vi "PH_PPPA_PowerUnit.PC_StateIgni.vi"(0 "i ref in":refnum<vi>, 3 "Igni Status":T1 items=["no info", "off/false/out", "on/true/in", "Failure", "Alarm", "Status 1", "Status 2", "Status 3"], 4 "not linked?":bool, 5 "error in (no error)":errorcluster) -> (14 "i ref out":refnum<vi>, 19 "error out":errorcluster)   [LabVIEW 2014, in "PH_PPPA_PowerUnit.lvlib"]
doc: "This VI writes the Ignitron Tag values to own attributes, calculates the state of the device and sets the GUI object."
uses:
  PH_PPPA_PowerUnit.lvlib
  PH_StatusHandler/PH_StatusHandler.Status.ctl
  PH_Common/PH_Common.lvlib
  PH_PowerUnit_BaseClass/PH_PowerUnit_BaseClass.lvlib
  PH_StatusHandler/PH_StatusHandler.lvlib
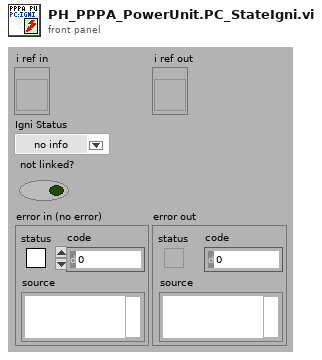
[diagram p1: front panel]
types:
  T1 = typedef "PH_StatusHandler.lvlib/PH_StatusHandler.Status.ctl" = i16
  T2 = typedef "PH_PPPA_PowerUnit.lvlib/PH_PPPA_PowerUnit.i attribute.ctl" = cluster{"GUI Refs":cluster{"Ignitron":refnum<vi>, "Rossrelais":refnum<vi>, "Set Voltage":refnum<vi>, "PSU":refnum<vi>, "EOC":refnum<vi>, "Trigger":refnum<vi>}, "Ignitron":T3, "PSU":T4, "Dump Ross Relais":T5, "Trigger":cluster{"State Device":T1, "linked?":bool}, "Timing Settings":cluster{"Prdc Fast?":bool, "Default Value Periodic Interval":i32, "Mercury on since":dbl, "Warm up Time Mercury [s]":dbl}, "Set Voltage [V]":dbl, "19er Ignitionbox":string}
  T3 = typedef "PH_PP_Common.lvlib/PH_PP_Common.Ignitron Attributes.ctl" = cluster{"State Device":T1, "linked?":bool}
  T4 = typedef "PH_PP_Common.lvlib/PH_PP_Common.PSU Attributes.ctl" = cluster{"lower limit [V]":dbl, "upper limit [V]":dbl, "Voltage set":bool, "State Device":T1, "linked?":bool}
  T5 = typedef "PH_PP_Common.lvlib/PH_PP_Common.Ross Relais Attributes.ctl" = cluster{"State Device":T1, "linked?":bool}
  T6 = typedef "PH_PowerUnit_BaseClass.lvlib/PH_PowerUnit_BaseClass.i attribute.ctl" = cluster{"Constructor finished":bool, "PU":cluster{"In use":bool, "Service ID in use":i32, "GUI Ref":refnum<vi>}, "Enabling":cluster{"State":T7, "GUI Ref":refnum<vi>}, "Timing":cluster{"Last Shot":dbl, "Time between Shots [Sec]":dbl, "Waiting Time over?":bool, "Service ID Waiting Time":i32, "GUI Ref":refnum<vi>, "Instance":cluster{"Status":T1, "linked?":bool, "GUI Ref":refnum<vi>}}, "Sequencer":cluster{"SM State":string, "GUI Ref":refnum<vi>, "linked":bool}, "Subscribed Trendmssgs":cluster{"Tagname":string, "Status":T1, "linked?":bool, "Shot Condition":T1, "GUI Ref":refnum<vi>}[], "PP PU":T8, "Default Voltage (V)":dbl, "GUI Refs":T9, "PSDB data":cluster{"Shot Voltage [V]":dbl, "State TO SM":T10, "Write 2 early":bool}, "State TO SM":T10}
  T7 = typedef "PH_SystemInformation.lvlib/PH_SystemInformationEnabling State.ctl" = i32
  T8 = typedef "PH_PP_Common.lvlib/PH_PP_Common.PUs.ctl" = enum16{"no Info", "PA-19mm-1", "PA-19mm-2", "PA-45mm-PILC", "PA-45mm-MAIN", "MA-PU-1", "MA-PU-2", "MA-PU-3", "MA-PU-4", "MA-PU-5", "MA-PU-6", "MA-FR", "MA-PILC", "PA-45mm-DP"}
  T9 = typedef "PH_PowerUnit_BaseClass.lvlib/PH_PowerUnit_BaseClass.GUI Refs.ctl" = cluster{"Delete Inst":refnum<vi>, "State TO SM":refnum<vi>, "State SM":refnum<vi>, "Fire":refnum<vi>}
  T10 = typedef "PH_PowerUnit_BaseClass.lvlib/PH_PowerUnit_BaseClass.SM States.ctl" = enum16{".", "Stand by", "Switch PU on", "Configure", "Set Default Voltage", "Set STANDBY", "Set READY", "Wait for Shot Cmd", "Open Dump Rods", "Open Ross Relais", "Close Ross Relais", "Switch PSU on", "Switch PSU off", "Charge", "Switch GD Channel on", "Close Dump Rods", "Rods-TO", "RR-TO", "PSU-TO", "Trigger-TO"}
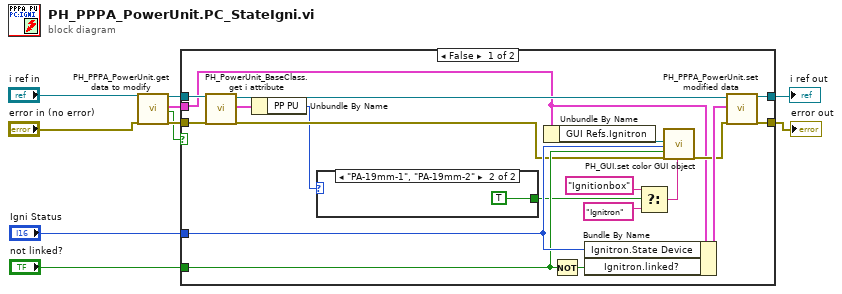
[diagram p0: block diagram]
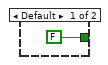
[diagram p2: hidden frame]
diagram:
  n1 = call "PH_PPPA_PowerUnit.get data to modify.vi"("i ref in"="i ref in", "error in (no error)"="error in (no error)") -> ("i ref out"=w10:refnum<vi>, "i attribute"=w8:T2, "timed out"=w7:bool, "error out"=w9:errorcluster)  [unwired: 14 in]
  n2 = case shown="False" w7 {
    tunnel: w10 -> [w23 w33]
    tunnel: [w18 w33] -> w4
    tunnel: w9 -> [w25 w32]
    tunnel: [w17 w32] -> w3
    tunnel: w8 -> [w13 _]
    tunnel: "Igni Status" -> [w28 _]
    tunnel: "not linked?" -> [w26 _]
    frame False {
      n3 = call "PH_PowerUnit_BaseClass.get i attribute.vi"("i ref in"=w23, "error in (no error)"=w25) -> ("i ref out"=w20:refnum<vi>, "i attribute"=w12:T6, "error out"=w24:errorcluster)  [unwired: 15 in]
      n4 = Unbundle By Name(w12) -> ("PP PU"=w11:T8)
      n5 = case shown="\"PA-19mm-1\", \"PA-19mm-2\"" w11 {
        tunnel: [FALSE TRUE] -> w16
        frame Default {
        }
        frame "PA-19mm-1", "PA-19mm-2" {
        }
      }
      n6 = Unbundle By Name(w13) -> ("GUI Refs.Ignitron"=w19:refnum<vi>)
      n7 = Not(x=w26) -> (.not. x?=w27:bool)
      n8 = Bundle By Name(cluster=w13, "Ignitron.State Device"=w28, "Ignitron.linked?"=w27) -> (w29:T2)
      n9 = Select(t="Ignitionbox", s=w16, f="Ignitron") -> (s? t:f=w14:string)
      n10 = call "PH_GUI.set color GUI object.vi"("GUI object Ref"=w19, "State"=w28, "Blinking? (false)"=w26, "error in (no error)"=w24, "Caption (N/A)"=w14) -> ("error out"=w15:errorcluster)  [unwired: 14 in]
      n11 = call "PH_PPPA_PowerUnit.set modified data.vi"("i ref in"=w20, "i attribute"=w29, "error in (no error)"=w15) -> ("i ref out"=w18:refnum<vi>, "error out"=w17:errorcluster)  [unwired: 15 in]
    }
    frame True {
    }
  }
  "error out" <- w3
  "i ref out" <- w4
